vi "GFITS_ArrList2StrList.vi"(9 "List In":string[][](table)) -> (2 "List Out":string)   [LabVIEW 2016]
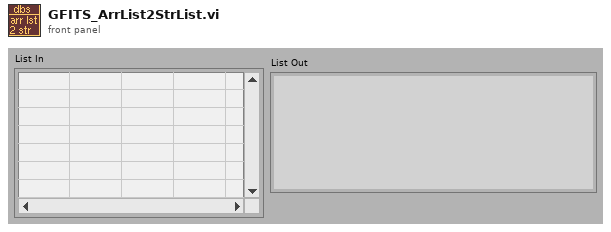
[diagram p1: front panel]
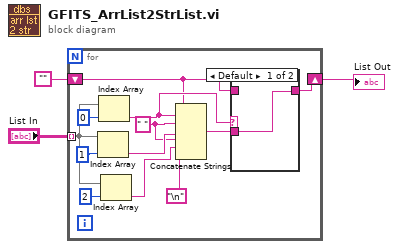
[diagram p0: block diagram]
diagram:
  n1 = for {
    tunnel: "List In" -> [w12] mode=indexing
    shift-right: [w5] -> w1
    shift-left: "" -> [w6]
    w10 = " " ("string")
    n2 = Index Array(array=w12, index=1) -> (element=w13:string)
    n3 = Index Array(array=w12, index=0) -> (element=w7:string)
    n4 = Index Array(array=w12, index=2) -> (element=w9:string)
    n5 = Concatenate Strings(w6, w7, w10, w13, w10, w9, "\n") -> (w4:string)
    n6 = case shown="Default" w7 {
      tunnel: w6 -> [_ w17]
      tunnel: [w16 w17] -> w5
      tunnel: w4 -> [w16 _]
      frame Default {
      }
      frame "", " " {
      }
    }
  }
  "List Out" <- w1
